vi "Query Calibration Date.vi"(0 "VISA resource name":refnum<visa-resource-name>, 11 "error IO":errorcluster) -> (3 "Date Format":enum16{"YMD", "MDY", "DMY"}(ring), 4 "VISA resource Out":refnum<visa-resource-name>, 6 "Day":i32 format="%02d", 8 "Month":i32 format="%02d", 10 "Year":i32 format="%02d", 15 "error Out":errorcluster)   [LabVIEW 2016, in "eec EST 300.lvlib"]
doc: "Returns the date the unit was last calibrated. It is recommended that you have this instrument recertified at least once per year."
uses:
  <instrlib>/eec EST 300/eec EST 300.lvlib
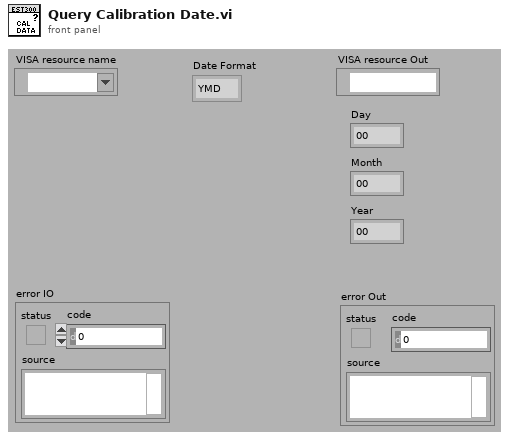
[diagram p1: front panel]
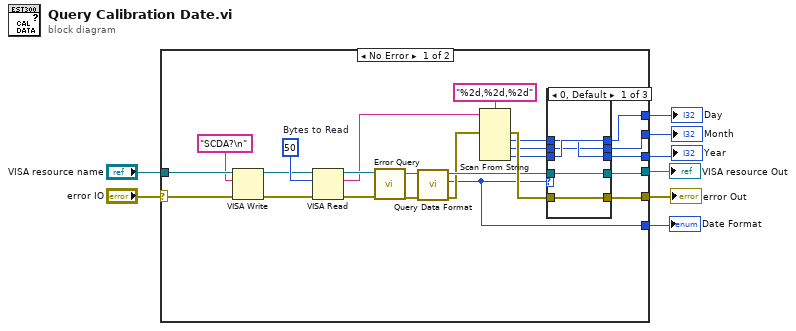
[diagram p0: block diagram]
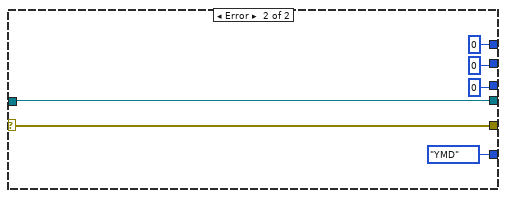
[diagram p4: hidden frame]
diagram:
  n1 = case shown="No Error" "error IO" {
    selector: "error IO" -> [w32 w53]
    tunnel: [w18 w53] -> w5
    tunnel: [w17 w52] -> w6
    tunnel: "VISA resource name" -> [w31 w52]
    tunnel: [w16 0] -> w4
    tunnel: [w15 0] -> w3
    tunnel: [w14 0] -> w2
    tunnel: [w9 enum16{"YMD", "MDY", "DMY"}."YMD" ("Date Format")] -> w1
    frame No Error {
      w29 = u32 50  # Bytes to Read
      n2 = VISA Write(VISA resource name=w31, write buffer="SCDA?\n" ("Command to Send (empty)"), error in (no error)=w32) -> (VISA resource name out=w26:refnum<visa-resource-name>, error out=w25:errorcluster)  [unwired: 1 out]
      n3 = VISA Read(VISA resource name=w26, byte count=w29, error in (no error)=w25) -> (VISA resource name out=w28:refnum<visa-resource-name>, read buffer=w19:string, error out=w27:errorcluster)  [unwired: 1 out]
      n4 = call <instrlib>:"Error Query.vi"("VISA resource name"=w28, "error in (no error)"=w27) -> ("VISA resource name out"=w12:refnum<visa-resource-name>, "error out"=w13:errorcluster)  [unwired: 10 in, 2 out]
      n5 = call <instrlib>:"Query Data Format.vi"("error IO"=w13, "VISA resource name"=w12) -> ("error Out"=w10:errorcluster, "Date Format"=w9:u16, "VISA resource Out"=w11:refnum<visa-resource-name>)  [unwired: 7 in]
      n6 = Scan From String(format string="%2d,%2d,%2d", input string=w19, error in=w10) -> (error out=w24:errorcluster, output 1=w21:i32, output 2=w22:i32, output 3=w23:i32)  [unwired: 4 in, 2 out]
      n7 = case shown="0, Default" w9 {
        tunnel: w11 -> [w34 w42 w44]
        tunnel: w24 -> [w33 w41 w43]
        tunnel: w21 -> [w36 w40 w47]
        tunnel: w22 -> [w35 w39 w46]
        tunnel: w23 -> [w37 w38 w45]
        tunnel: [w34 w42 w44] -> w17
        tunnel: [w33 w41 w43] -> w18
        tunnel: [w37 w39 w47] -> w16
        tunnel: [w35 w40 w46] -> w15
        tunnel: [w36 w38 w45] -> w14
        frame 0, Default {
        }
        frame 1 {
        }
        frame 2 {
        }
      }
    }
    frame Error {
    }
  }
  "VISA resource Out" <- w6
  "error Out" <- w5
  "Year" <- w2
  "Month" <- w3
  "Day" <- w4
  "Date Format" <- w1
